vi "Manage error firebase.vi"(8 "error in (no error)":errorcluster caption="entrée d'erreur (pas d'erreur)", 11 "Body":string) -> (0 "error out":errorcluster caption="sortie d'erreur")   [LabVIEW 2020, in "Library Instrument & Equipement.lvlib" / "Library FireBase.lvlib" / "Firebase Driver.lvclass"]
uses:
  Firebase Driver.lvclass
  JSON API/JSON Value/Set from JSON string.vi
  JSON API/JSON Value/JSON Value.lvclass
  Firebase Driver.lvclass/Firebase Driver.ctl
  JSON API/Variant JSON/Variant JSON.lvlib
  JSON API/Get Polymorphic/JSON GetSet.lvlib
panel:
  out "données":T1
  # "{\n  \"error\": {\n    \"code\": 429,\n    \"message\": \"Quota exceeded.\",\n    \"status\": \"RESOURCE_EXHAUSTED\"\n  }\n}"
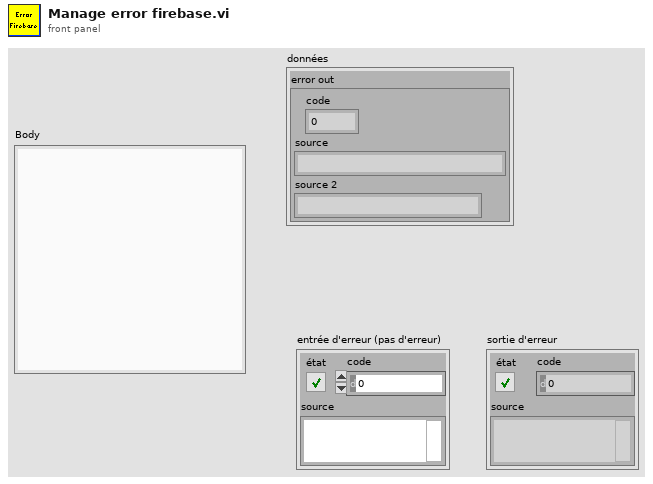
[diagram p1: front panel]
types:
  T1 = cluster{"error out":cluster{"code":i32, "source":string, "source 2":string}}
  T2 = cluster{"error":cluster{"code":i32, "message":string, "status":string}}
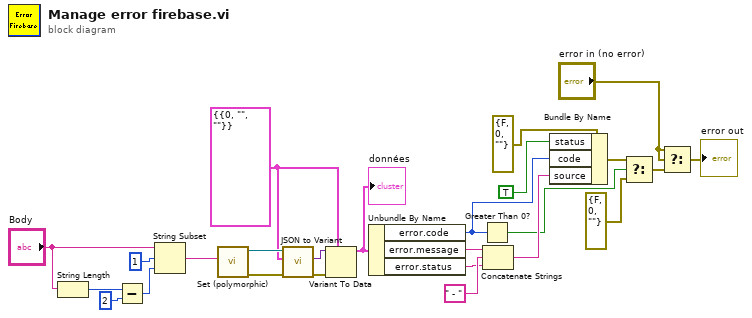
[diagram p0: block diagram]
diagram:
  w21 = T2 {"error"={"code"=0, "message"="", "status"=""}} ("Cluster")
  n1 = String Length(string="Body") -> (length=w5:i32)
  n2 = Subtract(x=w5, y=2) -> (x-y=w3:i32)
  n3 = String Subset(string="Body", offset (0)=1, length (rest)=w3) -> (substring=w1:string)
  n4 = call-poly "Set (polymorphic).vi"("JSON stream"=w1) -> ("error out"=w22:errorcluster, "JSON Value out"=w25:refnum<class "JSON Value.lvclass">)  [unwired: 8 in, 1 out]
  n5 = call "JSON to Variant.vi"("error in (no error)"=w22, "Variant (Data Type)"=w21, "JSON Value"=w25) -> ("error out"=w23:errorcluster, "Variant out"=w24:variant)  [unwired: 7 in]
  n6 = Variant To Data(error in=w23, type=w21, Variant=w24) -> (data=w20:T2)  [unwired: 1 out]
  "données" <- w20
  n7 = Unbundle By Name(w20) -> ("error.code"=w10:i32, "error.message"=w15:string, "error.status"=w13:string)
  n8 = Greater Than 0?(x=w10) -> (x > 0?=w9:bool)
  n9 = Concatenate Strings(w15, " - " ("chaîne"), w13) -> (w12:string)
  n10 = Bundle By Name(cluster=errorcluster {"status"=FALSE, "code"=0, "source"=""} ("error in (no error)"), "status"=TRUE, "code"=w10, "source"=w12) -> (w11:errorcluster)
  n11 = Select(t=w11, s=w9, f=errorcluster {"status"=FALSE, "code"=0, "source"=""} ("cas faux")) -> (s? t:f=w7:errorcluster)
  n12 = Select(t="error in (no error)", s="error in (no error)", f=w7) -> (s? t:f=→"error out":errorcluster)
